vi "GetAttributeViInt32_ACP_CL_DD.vi"(8 "error in (no error)":errorcluster {"code" format="%.0x"}, 9 "AttributeID":u32(ring)=1191759 items=["DIGITAL_DEMOD_AVERAGE_COUNT"=1191759, "DIGITAL_DEMOD_AVERAGE_MODE"=1191757, "DIGITAL_DEMOD_CPM_INDEX"=1191642, "DIGITAL_DEMOD_DISPLAY_BITS_FORMAT"=1191625, "DIGITAL_DEMOD_DISPLAY_IDEAL_STATE_SHAPE"=1191615, "DIGITAL_DEMOD_DISPLAY_VIEW_SELECTION"=1191588, "DIGITAL_DEMOD_DISPLAY_WINDOW_TRACE_DATA_FORMAT"=1191665, "DIGITAL_DEMOD_DISPLAY_WINDOW_TRACE_DATA_TYPE"=1191666, "DIGITAL_DEMOD_DISPLAY_WINDOW_X_REF_POSITION"=1191610, "DIGITAL_DEMOD_DISPLAY_WINDOW_X_TIME_UNIT"=1191614, "DIGITAL_DEMOD_DISPLAY_WINDOW_Y_POSITION"=1191592, "DIGITAL_DEMOD_EQUALIZATION_FILTER_LENGTH"=1191634, "DIGITAL_DEMOD_EVM_NORMALIZATION_REFERENCE"=1191667, "DIGITAL_DEMOD_FILTER_REFERENCE"=1191630, "DIGITAL_DEMOD_FILTER_TYPE"=1191627, "DIGITAL_DEMOD_LIMITS_CLOCK_ERROR_UNIT"=1191620, "DIGITAL_DEMOD_LIMITS_FREQUENCY_ERROR_UNIT"=1191621, "DIGITAL_DEMOD_MARKER_ACTIVE_MARKER"=1191593, "DIGITAL_DEMOD_MARKER_COUNT"=1191595, "DIGITAL_DEMOD_MARKER_DELTA_REFERENCE"=1191596, "DIGITAL_DEMOD_MARKER_FUNCTION"=1191607, "DIGITAL_DEMOD_MARKER_TYPE"=1191601, "DIGITAL_DEMOD_MODULATION_FORMAT"=1191637, "DIGITAL_DEMOD_PHASE_NOISE_OPTIMIZATION"=1191660, "DIGITAL_DEMOD_POINTS_PER_SAMPLE"=1191626, "DIGITAL_DEMOD_SWEEPCOUPLING_SWEEP_POINTS"=1191765, "DIGITAL_DEMOD_SYNC_OFFSET"=1191650, "DIGITAL_DEMOD_TRACE_COUNT"=1191661, "DIGITAL_DEMOD_TRACE_LIMIT_COUNT"=1191668, "DIGITAL_DEMOD_TRACE_LIMIT_TYPE"=1191676, "DIGITAL_DEMOD_TRACE_LIMIT_WINDOW_LIMIT"=1191678, "DIGITAL_DEMOD_TRACE_LIMIT_X_REFERENCE"=1191677, "DIGITAL_DEMOD_TRACE_LIMIT_X_UNIT"=1191672, "DIGITAL_DEMOD_TRACE_LIMIT_Y_UNIT"=1191761, "DIGITAL_DEMOD_TRIGGER_SOURCE"=1191613, "DIGITAL_DEMOD_WINDOW_COUNT"=1191756, "FFT_WINDOW"=1191766, "GATING_DELAY_COMPENSATION"=1150141, "GATING_SOURCE"=1190018, "GATING_TYPE"=1190019, "INPUT_IQ_FEED_TYPE"=1190844, "INPUT_IQ_I_COUPLING"=1191695, "INPUT_IQ_I_IMPEDANCE"=1191701, "INPUT_IQ_IMPEDANCE"=1191699, "INPUT_IQ_Q_COUPLING"=1191696, "INPUT_IQ_Q_IMPEDANCE"=1191702, "INPUT_RF_PRE_AMPLIFIER_BAND"=1190118, "LEVEL_ATTENUATION_OPTIMIZE"=1190119, "LEVEL_ATTENUATION_STEP_INCREMENT"=1190120], 10 "RepCapIdentifier":string, 11 "instrument handle":refnum<k15>) -> (0 "error out":errorcluster {"code" format="%.0x"}, 2 "AttributeValue":i32, 3 "instrument handle out":refnum<k15>)   [LabVIEW 2021, in "Keysight XSAnVMA.lvlib"]
doc: "Gets Int32 Attribute from instrumrnt driver.\nThe following attributes are supported:\n\nACP_AVERAGE_COUNT\nACP_AVERAGE_MODE\nACP_CARRIER_COUNT\nACP_CARRIER_POWER_REFERENCE_TYPE\nACP_CARRIER_REFERENCE_NUMBER\nACP_DETECTOR_TYPE\nACP_DISPLAY_VIEW_SELECTION\nACP_DISPLAY_WINDOWY_REF_POSITION\nACP_FAST_POWER_IF_GAIN\nACP_FAST_POWER_RBW_MODE\nACP_FREQUENCY_PHASE_NOISE_OPTION_STATE\nACP_MARKER_ACTIVE_MARKER\nACP_MARKER_COUNT\nACP_MARKER_DELTA_REFERENCE\nACP_MARKER_TRACE\nACP_MARKER_TYPE\nACP_MEASUREMENT_METHOD\nACP_MEASUREMENT_TYPE\nACP_POWER_SPECTRAL_DENSITY_REFERENCE\nACP_SWEEPCOUPLING_BANDWIDTH_SHAPE\nACP_SWEEPCOUPLING_BANDWIDTH_TYPE\nACP_SWEEPCOUPLING_SWEEP_POINTS\nACP_SWEEPCOUPLING_SWEEP_TIME_AUTO_RULES\nACP_TRACE_COUNT\nACP_TRIGGER_SOURCE\nANALOG_ANTI_ALIASING_FILTER_TYPE\nDIGITAL_DEMOD_AVERAGE_COUNT\nDIGITAL_DEMOD_AVERAGE_MODE\nDIGITAL_DEMOD_CPM_INDEX\nDIGITAL_DEMOD_DISPLAY_BITS_FORMAT\nDIGITAL_DEMOD_DISPLAY_IDEAL_STATE_SHAPE\nDIGITAL_DEMOD_DISPLAY_VIEW_SELECTION\nDIGITAL_DEMOD_DISPLAY_WINDOW_TRACE_DATA_FORMAT\nDIGITAL_DEMOD_DISPLAY_WINDOW_TRACE_DATA_TYPE\nDIGITAL_DEMOD_DISPLAY_WINDOW_X_REF_POSITION\nDIGITAL_DEMOD_DISPLAY_WINDOW_X_TIME_UNIT\nDIGITAL_DEMOD_DISPLAY_WINDOW_Y_POSITION\nDIGITAL_DEMOD_EQUALIZATION_FILTER_LENGTH\nDIGITAL_DEMOD_EVM_NORMALIZATION_REFERENCE\nDIGITAL_DEMOD_FILTER_REFERENCE\nDIGITAL_DEMOD_FILTER_TYPE\nDIGITAL_DEMOD_LIMITS_CLOCK_ERROR_UNIT\nDIGITAL_DEMOD_LIMITS_FREQUENCY_ERROR_UNIT\nDIGITAL_DEMOD_MARKER_ACTIVE_MARKER\nDIGITAL_DEMOD_MARKER_COUNT\nDIGITAL_DEMOD_MARKER_DELTA_REFERENCE\nDIGITAL_DEMOD_MARKER_FUNCTION\nDIGITAL_DEMOD_MARKER_TYPE\nDIGITAL_DEMOD_MODULATION_FORMAT\nDIGITAL_DEMOD_PHASE_NOISE_OPTIMIZATION\nDIGITAL_DEMOD_POINTS_PER_SAMPLE\nDIGITAL_DEMOD_SWEEPCOUPLING_SWEEP_POINTS\nDIGITAL_DEMOD_SYNC_OFFSET\nDIGITAL_DEMOD_TRACE_COUNT\nDIGITAL_DEMOD_TRACE_LIMIT_COUNT\nDIGITAL_DEMOD_TRACE_LIMIT_TYPE\nDIGITAL_DEMOD_TRACE_LIMIT_WINDOW_LIMIT\nDIGITAL_DEMOD_TRACE_LIMIT_X_REFERENCE\nDIGITAL_DEMOD_TRACE_LIMIT_X_UNIT\nDIGITAL_DEMOD_TRACE_LIMIT_Y_UNIT\nDIGITAL_DEMOD_TRIGGER_SOURCE\nDIGITAL_DEMOD_WINDOW_COUNT\nFFT_WINDOW\nGATING_DELAY_COMPENSATION\nGATING_SOURCE\nGATING_TYPE\nINPUT_IQ_FEED_TYPE\nINPUT_IQ_I_COUPLING\nINPUT_IQ_I_IMPEDANCE\nINPUT_IQ_IMPEDANCE\nINPUT_IQ_Q_COUPLING\nINPUT_IQ_Q_IMPEDANCE\nINPUT_RF_PRE_AMPLIFIER_BAND\nLEVEL_ATTENUATION_OPTIMIZE\nLEVEL_ATTENUATION_STEP_INCREMENT"
uses:
  <instrlib>/Keysight XSAnVMA/Keysight XSAnVMA.lvlib
  KtXSAnVMA_64.dll
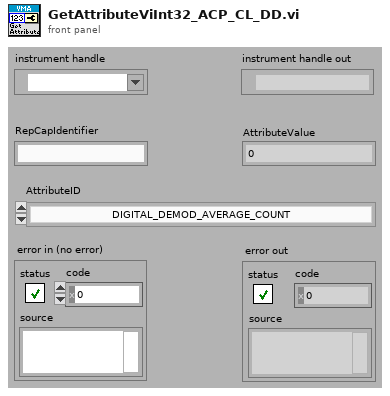
[diagram p1: front panel]
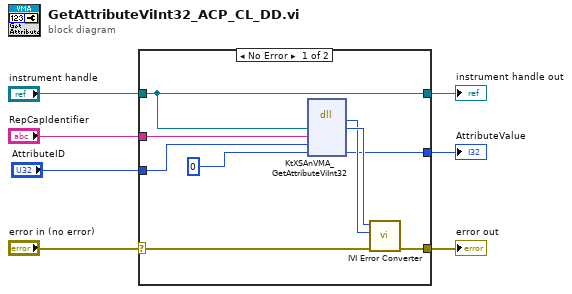
[diagram p0: block diagram]
diagram:
  n1 = case shown="No Error" "error in (no error)" {
    selector: "error in (no error)" -> [w14 w18]
    tunnel: [w13 w18] -> w7
    tunnel: "instrument handle" -> [w8 w17]
    tunnel: "RepCapIdentifier" -> [w12 _]
    tunnel: "AttributeID" -> [w11 _]
    tunnel: [w9 _] -> w3
    tunnel: [w8 w17] -> w2
    frame No Error {
      n2 = dll-call lib="KtXSAnVMA**.dll" fn="KtXSAnVMA_GetAttributeViInt32"("Vi"=w8, "RepCapIdentifier"=w12, "AttributeID"=w11, "AttributeValue"=0) -> ("return type"=w15:i32, "Vi"=w16:u32, "AttributeValue"=w9:i32)  [unwired: 5 in, 2 out]
      n3 = call <instrlib>:"IVI Error Converter.vi"("error in (no error)"=w14, "IVI error code (0)"=w15, "instrument handle"=w16) -> ("error out"=w13:errorcluster)  [unwired: 7 in, 1 out]
    }
    frame Error {
    }
  }
  "error out" <- w7
  "instrument handle out" <- w2
  "AttributeValue" <- w3
